vi "rad_ConvertImageFiles.vi"(4 "error in":errorcluster, 5 "ImageFiles":string[](array[string]), 7 "ImageFolderRoot":path) -> (0 "error out":errorcluster)   [LabVIEW 2020]
uses:
  <userlib>/_OpenG.lib/lvzip/lvzip.llb/subVI/ZLIB Extract All Files To Dir (Path)__ogtk.vi
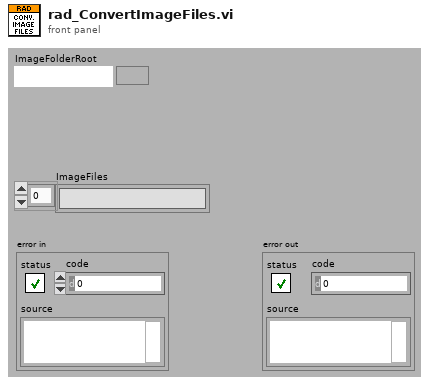
[diagram p1: front panel]
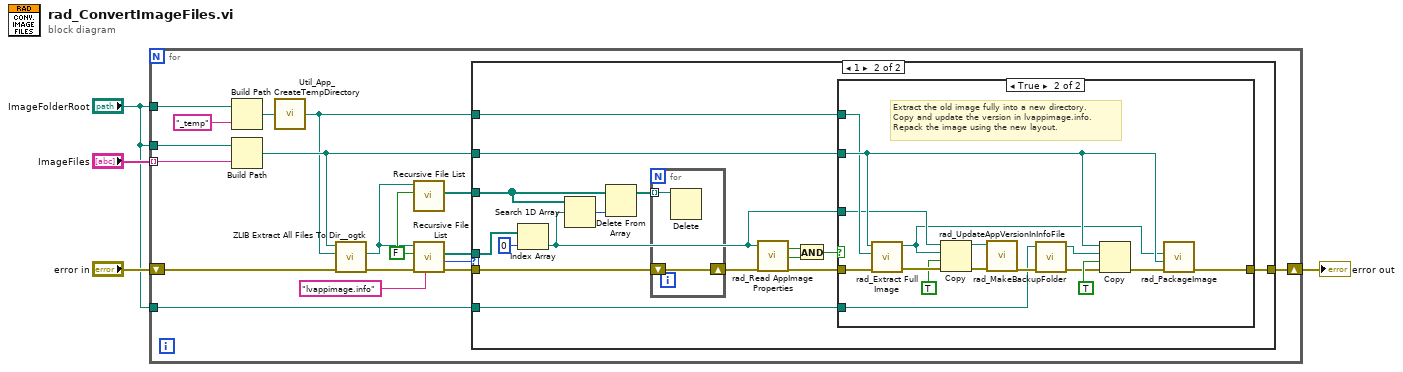
[diagram p0: block diagram]
diagram:
  n1 = for {
    tunnel: "ImageFiles" -> [w16] mode=indexing
    tunnel: "ImageFolderRoot" -> [w21]
    tunnel: "ImageFolderRoot" -> [w20]
    shift-right: [w19] -> w4
    shift-left: "error in" -> [w14]
    tunnel: "ImageFolderRoot" -> [w17]
    w9 = FALSE ("Treat LLBs as Folders?")
    n2 = Build Path(base path=w21, name or relative path="_temp") -> (appended path=w18:path)
    n3 = Build Path(base path=w17, name or relative path=w16) -> (appended path=w15:path)
    n4 = call "Util_App_CreateTempDirectory.vi"("TempFolderPath"=w18) -> ("TempFolderPath_out"=w13:path)
    n5 = call-poly <userlib>:"ZLIB Extract All Files To Dir__ogtk.vi"("error in (no error)"=w14, "destination directory (archive name without ending)"=w13, "archive name (file dialog)"=w15) -> ("error out"=w12:errorcluster, "destination directory out"=w8:path)  [unwired: 6 in, 1 out]
    n6 = call <vilib>:"Recursive File List.vi"("Treat LLBs as Folders?"=w9, "Folder Path"=w8) -> ("All Files in Dir"=w5:path[])  [unwired: 5 in, 4 out]
    n7 = call <vilib>:"Recursive File List.vi"("pattern"="lvappimage.info", "error in (no error)"=w12, "Treat LLBs as Folders?"=w9, "Folder Path"=w8) -> ("error out"=w11:errorcluster, "Number of Files"=w6:i32, "All Files in Dir"=w7:path[])  [unwired: 3 in, 2 out]
    n8 = case shown="1" w6 {
      tunnel: w20 -> [_ w35]
      tunnel: [_ w34] -> w19
      tunnel: w15 -> [_ w31]
      tunnel: w13 -> [_ w30]
      tunnel: w11 -> [_ w24]
      tunnel: w7 -> [_ w29]
      tunnel: w5 -> [_ w27]
      frame Default {
      }
      frame 1 {
        n9 = Index Array(array=w29, index=0) -> (element=w28:path)
        n10 = Search 1D Array(1D array=w27, element=w28) -> (index of element=w26:i32)  [unwired: 1 in]
        n11 = Delete From Array(array=w27, index=w26) -> (array with subset deleted=w23:path[])  [unwired: 1 in, 1 out]
        n12 = for {
          shift-right: [w40] -> w25
          shift-left: w24 -> [w40]
          tunnel: w23 -> [w39] mode=indexing
          n13 = Delete(path (use dialog)=w39) -> ()  [unwired: 4 in, 3 out]
        }
        n14 = call "rad_Read AppImage Properties.vi"("AppImage Properties Path"=w28, "error in (no error)"=w25) -> ("Supported"=w38:bool, "Older"=w37:bool, "error out"=w33:errorcluster)  [unwired: 12 in, 3 out]
        n15 = And(x=w38, y=w37) -> (x .and. y?=w36:bool)
        n16 = case shown="True" w36 {
          tunnel: w31 -> [_ w49]
          tunnel: w30 -> [_ w48]
          tunnel: w35 -> [_ w53]
          tunnel: [w41 w51] -> w34
          tunnel: w33 -> [w41 w50]
          tunnel: w28 -> [_ w45]
          frame False {
          }
          frame True {
            # "Extract the old image fully into a new directory.\nCopy and update the version in lvappimage.info.\nRepack the image using the new layout."
            n17 = call "rad_Extract Full Image.vi"("error in (no error)"=w50, "App Image Temp Folder"=w48, "Zipped App Image File Path"=w49) -> ("error out"=w47:errorcluster, "Unzipped App Image Folder Path"=w44:path)  [unwired: 7 in]
            n18 = Copy(8:w47, 9:TRUE ("overwrite (F)"), 10:w44, 11:w45) -> (0:w46:errorcluster, 3:w43:path)  [unwired: 1 in, 1 out]
            n19 = call "rad_UpdateAppVersionInInfoFile.vi"("error in"=w46, "Path to lvappimage.info"=w43) -> ("error out"=w56:errorcluster)  [unwired: 9 in]
            n20 = call "rad_MakeBackupFolder.vi"("error in"=w56, "ImagePathFolder"=w53) -> ("error out"=w55:errorcluster, "BackupFolderPath"=w54:path)  [unwired: 2 in]
            n21 = Copy(8:w55, 9:TRUE ("overwrite (F)"), 10:w54, 11:w49) -> (0:w52:errorcluster)  [unwired: 1 in, 2 out]
            n22 = call "rad_PackageImage.vi"("error in (no error)"=w52, "AppImage Path"=w49, "Temp Image Path"=w44) -> ("error out"=w51:errorcluster)  [unwired: 8 in]
          }
        }
      }
    }
  }
  "error out" <- w4
